vi "VASP Janitor.vi"() -> ()   [LabVIEW 2010]
uses:
  <vilib>/Utility/error.llb/DialogType.ctl
  <vilib>/addons/database/Connection.llb/DB Tools Open Connec (Path).vi
  <vilib>/addons/database/NI_Database_API.lvlib
  <vilib>/addons/database/Connection.llb/Conn Execute.vi
  <vilib>/addons/database/Recordset.llb/Rec Destroy - Connection.vi
panel:
  in  "Tab Control 2":enum32{"File Uploader", "Backup"}(tab)
  in  "Delete Old?":bool=TRUE
  in  "Primary Path":path=path "D:/Ab-initio/VASP Calcs/2D_Grain Boundaries"
  in  "Compress?":bool=TRUE
  in  "Time Between Uploads (min)":dbl=15.0
  in  "Next Upload Time":timestamp=timestamp(3475418756.730113 s since 1904-01-01) format="%<%I:%M:%S %p>T"
  out "Current Time":string="11:50:58 AM"
  in  "Upload Now":bool
  out "Status":string="Opening Connection to Database"
  out "Uploading":bool=TRUE
  in  "Supress Upload Errors":bool
  in  "Compressed File Type":string(combo)="7z"
  in  "Periodic Database Backup":bool=TRUE
  out "Last DB Backup":timestamp=timestamp(3394540298 s since 1904-01-01)
  out "x-y":dbl
  in  "UDL Path":path=path "D:/Ab-initio/VASP Calcs/VASP DB.udl"
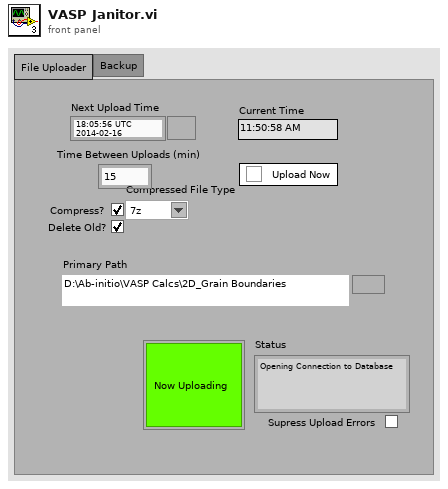
[diagram p1: front panel]
types:
  T1 = typedef "NI_Database_API.lvlib/Conn ObjectReference.ctl" = refnum<k1>
  T2 = typedef "DialogType.ctl" = u16
  T3 = enum16{"Left Button", "Center Button", "Right Button", "Window Close"}
  T4 = typedef "NI_Database_API.lvlib/Rec ObjectReference.ctl" = refnum<k1>
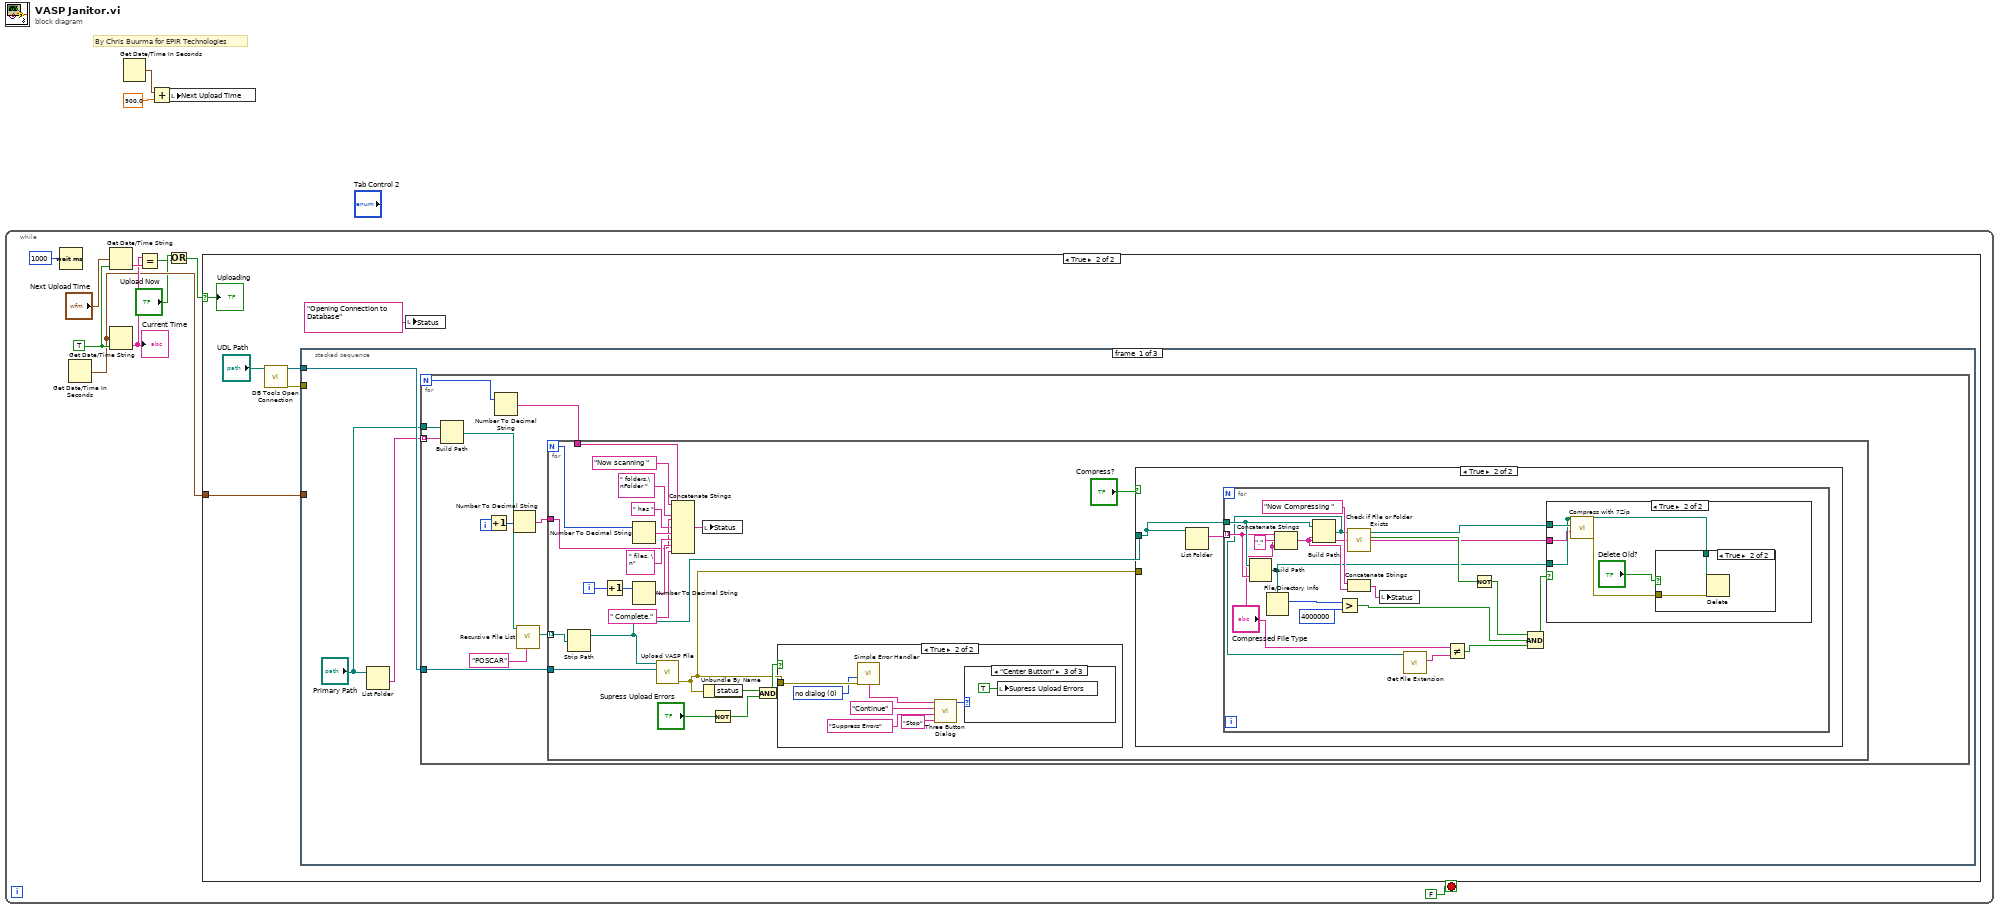
[diagram p0: block diagram]
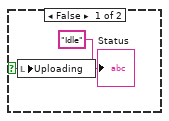
[diagram p2: hidden frame]
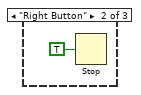
[diagram p8: hidden frame]
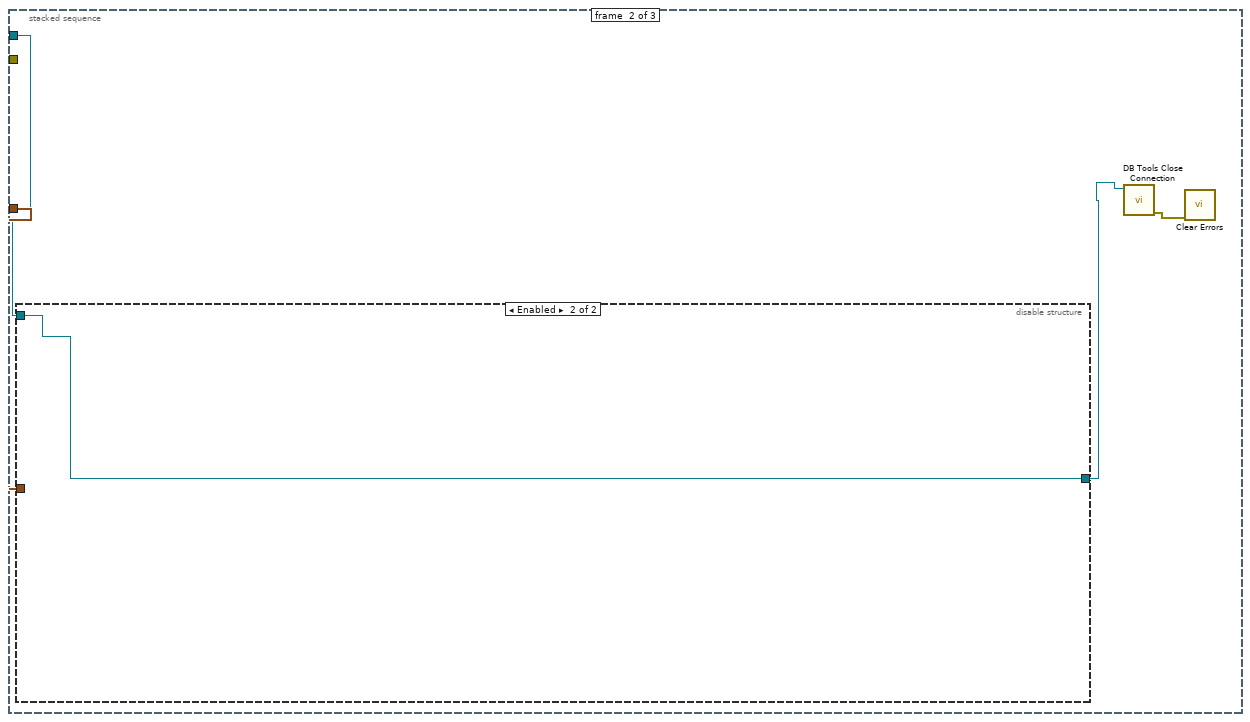
[diagram p9: hidden frame]
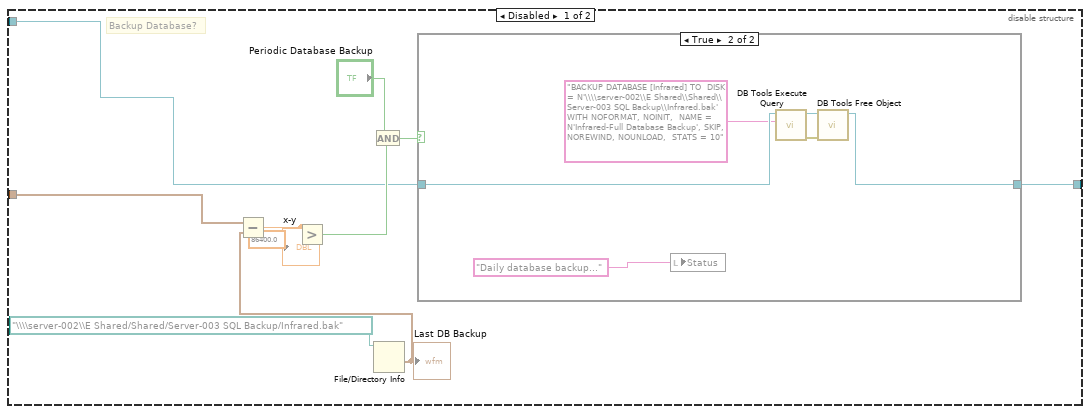
[diagram p10: hidden frame]
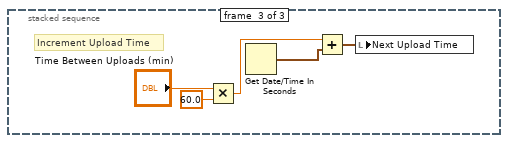
[diagram p12: hidden frame]
diagram:
  # "By Chris Buurma for EPIR Technologies"
  n1 = while {
    stop <- FALSE stop-if-true
    w8 = TRUE ("want seconds? (F)")
    n2 = Wait (ms)(milliseconds to wait=u32 1000) -> ()  [unwired: 1 out]
    n3 = Get Date/Time In Seconds() -> (seconds since 1Jan1904=w7:timestamp)
    n4 = Get Date/Time String(seconds (now)="Next Upload Time", want seconds? (F)=w8) -> (time string=w10:string)  [unwired: 1 in, 1 out]
    n5 = Get Date/Time String(seconds (now)=w7, want seconds? (F)=w8) -> (time string=w9:string)  [unwired: 1 in, 1 out]
    "Current Time" <- w9
    n6 = Equal?(x=w9, y=w10) -> (x = y?=w5:bool)
    n7 = Or(x="Upload Now", y=w5) -> (x .or. y?=w4:bool)
    n8 = case shown="True" w4 {
      selector: w4 -> [w15 w21]
      tunnel: w7 -> [_ w20]
      frame False {
        n9 = local write "Uploading"(w15) -> ()
        "Status" <- "Idle" ("Status")
      }
      frame True {
        n10 = call-poly <vilib>:"DB Tools Open Connection.vi"("connection information"="UDL Path") -> ("error out"=w16:errorcluster, "connection reference"=w18:T1)  [unwired: 7 in]
        n11 = stacked-sequence {
          tunnel: w20 -> [_ w97 _]
          tunnel: w18 -> [w24 w96 _]
          tunnel: w16 -> [_ _ _]
          frame #0 {
            n12 = List Folder(path="Primary Path") -> (folder names=w23:string[])  [unwired: 3 in, 3 out]
            n13 = for {
              N -> [w29]
              tunnel: w24 -> [w35]
              tunnel: w23 -> [w33] mode=indexing
              tunnel: "Primary Path" -> [w34]
              i -> [w26]
              n14 = Build Path(base path=w34, name or relative path=w33) -> (appended path=w30:path)
              n15 = Increment(x=w26) -> (x+1=w25:i32)
              n16 = Number To Decimal String(number=w29) -> (decimal integer string=w28:string)  [unwired: 1 in]
              n17 = Number To Decimal String(number=w25) -> (decimal integer string=w27:string)  [unwired: 1 in]
              n18 = call <vilib>:"Recursive File List.vi"("pattern"="POSCAR", "Folder Path"=w30) -> ("All Files in Dir"=w31:path[])  [unwired: 5 in, 4 out]
              n19 = for {
                N -> [w53]
                tunnel: w35 -> [w46]
                tunnel: w31 -> [w45] mode=indexing
                tunnel: w28 -> [w44]
                tunnel: w27 -> [w42]
                i -> [w40]
                n20 = Strip Path(path=w45) -> (stripped path=w36:path)  [unwired: 1 out]
                n21 = Increment(x=w40) -> (x+1=w39:i32)
                n22 = Number To Decimal String(number=w53) -> (decimal integer string=w57:string)  [unwired: 1 in]
                n23 = Number To Decimal String(number=w39) -> (decimal integer string=w52:string)  [unwired: 1 in]
                n24 = call "Upload VASP File.vi"("connection reference"=w46, "Directory to upload"=w36) -> ("error out"=w37:errorcluster)  [unwired: 8 in, 1 out]
                n25 = Concatenate Strings("Now scanning " ("string"), w44, " folders.\nFolder " ("string"), w42, " has " ("string"), w57, " files. \n" ("string"), w52, " Complete." ("string")) -> (w54:string)
                n26 = local write "Status"(w54) -> ()
                n27 = Unbundle By Name(w37) -> ("status"=w50:bool)
                n28 = Not(x="Supress Upload Errors") -> (.not. x?=w49:bool)
                n29 = And(x=w50, y=w49) -> (x .and. y?=w47:bool)
                n30 = case shown="True" w47 {
                  tunnel: w37 -> [_ w91]
                  frame False {
                  }
                  frame True {
                    w90 = T2 0 items=["no dialog", "OK message", "continue or stop message", "OK message + warnings", "continue/stop + warnings"] ("type of dialog (OK msg:1)")
                    n31 = call <vilib>:"Simple Error Handler.vi"("type of dialog (OK msg:1)"=w90, "error in (no error)"=w91) -> ("message"=w89:string)  [unwired: 3 in, 4 out]
                    n32 = call <vilib>:"Three Button Dialog.vi"("Right Button Text (\"Cancel\")"="Stop" ("Right Button Text (\"Cancel\")"), "Center Button Text (\"No\")"="Suppress Errors" ("F button name (\"Cancel\")"), "Left Button Text (\"Yes\")"="Continue" ("Left Button Text (\"Yes\")"), "message"=w89) -> ("Which Button?"=w85:T3)  [unwired: 7 in]
                    n33 = case shown="\"Center Button\"" w85 {
                      frame "Left Button", Default {
                      }
                      frame "Right Button" {
                        n34 = Stop(stop? (T)=TRUE) -> ()
                      }
                      frame "Center Button" {
                        n35 = local write "Supress Upload Errors"(TRUE ("Supress Upload Errors")) -> ()
                      }
                    }
                  }
                }
                n36 = case shown="True" "Compress?" {
                  tunnel: w37 -> [_ _]
                  tunnel: w36 -> [_ w58]
                  frame False {
                  }
                  frame True {
                    n37 = List Folder(path=w58) -> (filenames=w59:string[])  [unwired: 3 in, 3 out]
                    n38 = for {
                      tunnel: w58 -> [w72]
                      tunnel: w59 -> [w71] mode=indexing
                      n39 = Build Path(base path=w72, name or relative path=w71) -> (appended path=w67:path)
                      n40 = File/Directory Info(path=w67) -> (size=w70:i64)  [unwired: 1 in, 6 out]
                      n41 = Concatenate Strings(w71, "." ("string"), "Compressed File Type") -> (w73:string)
                      n42 = Build Path(base path=w72, name or relative path=w73) -> (appended path=w60:path)
                      n43 = Greater?(x=w70, y=i64 4000000) -> (0:w66:bool)
                      n44 = call <vilib>:"Check if File or Folder Exists.vi"("path"=w60) -> ("file or folder exists?"=w69:bool, "dup path"=w76:path)  [unwired: 8 in, 1 out]
                      n45 = Concatenate Strings("Now Compressing " ("Status"), w73) -> (w74:string)
                      n46 = local write "Status"(w74) -> ()
                      n47 = call <vilib>:"Get File Extension.vi"("file"=w60) -> ("lowercase file extension"=w63:string)  [unwired: 7 in, 3 out]
                      n48 = Not Equal?(x="Compressed File Type", y=w63) -> (x != y?=w62:bool)
                      n49 = Not(x=w69) -> (.not. x?=w65:bool)
                      n50 = Compound Arithmetic op=AND(w65, w66, w62) -> (w61:bool)
                      n51 = case shown="True" w61 {
                        tunnel: w67 -> [_ w79]
                        tunnel: w76 -> [_ w82]
                        tunnel: "Compressed File Type" -> [_ w78]
                        frame False {
                        }
                        frame True {
                          n52 = call "Compress with 7Zip.vi"("Compressed File Type"=w78, "7z File to compress into"=w82, "Folder or file to compress"=w79) -> ("error out"=w80:errorcluster)  [unwired: 8 in]
                          n53 = case shown="True" "Delete Old?" {
                            tunnel: w80 -> [_ w84]
                            tunnel: w79 -> [_ w83]
                            frame False {
                            }
                            frame True {
                              n54 = Delete(path (use dialog)=w83, error in=w84) -> ()  [unwired: 3 in, 3 out]
                            }
                          }
                        }
                      }
                    }
                  }
                }
              }
            }
          }
          frame #1 {
            n55 = disable-structure shown="Enabled" {
              disable-tunnel: w97 -> [w105 _]
              disable-tunnel: w96 -> [w100 w115]
              disable-tunnel: [w99 w115] -> w95
              frame Disabled {
                # "Backup Database?"
                n56 = File/Directory Info(path=path "\\\\server-002\\E Shared/Shared/Server-003 SQL Backup/Infrared.bak" ("Path")) -> (last mod=w104:timestamp)  [unwired: 1 in, 6 out]
                "Last DB Backup" <- w104
                n57 = Subtract(x=w105, y=w104) -> (x-y=w103:dbl)
                "x-y" <- w103
                n58 = Greater?(x=w103, y=86400.0) -> (0:w102:bool)
                n59 = And(x="Periodic Database Backup", y=w102) -> (x .and. y?=w98:bool)
                n60 = case shown="True" w98 {
                  tunnel: w100 -> [w108 w112]
                  tunnel: [w108 w113] -> w99
                  frame False {
                  }
                  frame True {
                    n61 = local write "Status"("Daily database backup..." ("Status")) -> ()
                    n62 = call-poly <vilib>:"DB Tools Execute Query.vi"("SQL query"="BACKUP DATABASE [Infrared] TO  DISK = N'\\\\server-002\\E Shared\\Shared\\Server-003 SQL Backup\\Infrared.bak' WITH NOFORMAT, NOINIT,  NAME = N'Infrared-Full Database Backup', SKIP, NOREWIND, NOUNLOAD,  STATS = 10", "connection reference"=w112) -> ("error out"=w110:errorcluster, "recordset reference"=w114:T4)  [unwired: 6 in]
                    n63 = call-poly <vilib>:"DB Tools Free Object.vi"("error in (no error)"=w110, "recordset reference"=w114) -> ("connection reference"=w113:T1)  [unwired: 8 in, 1 out]
                  }
                }
              }
              frame Enabled {
              }
            }
            n64 = call <vilib>:"DB Tools Close Connection.vi"("connection reference"=w95) -> ("error out"=w94:errorcluster)  [unwired: 6 in]
            n65 = call <vilib>:"Clear Errors.vi"("error in (no error)"=w94) -> ()  [unwired: 6 in, 1 out]
          }
          frame #2 {
            # "Increment Upload Time"
            n66 = Multiply(x="Time Between Uploads (min)", y=60.0) -> (x*y=w119:dbl)
            n67 = Get Date/Time In Seconds() -> (seconds since 1Jan1904=w116:timestamp)
            n68 = Add(x=w119, y=w116) -> (x+y=w120:timestamp)
            n69 = local write "Next Upload Time"(w120) -> ()
          }
        }
        n70 = local write "Status"("Opening Connection to Database" ("Status")) -> ()
        "Uploading" <- w21
      }
    }
  }
  n71 = Get Date/Time In Seconds() -> (seconds since 1Jan1904=w3:timestamp)
  n72 = Add(x=w3, y=900.0) -> (x+y=w1:timestamp)
  n73 = local write "Next Upload Time"(w1) -> ()
